vi "Install Project.vi"() -> ()   [LabVIEW 2011, in "LVH-Toolbox.lvlib" / "LVH-Build-Tools.lvlib"]
doc: "This VI will copy the source files into the install directory and create hard links replace the source files with hard links to the install directory.\n\nNote: Do not open any VI's from the source directory. All edits should be done in the Install directory to preserve paths."
uses:
  LVH-Build-Tools.lvlib
  Private/Type Defs/Install State.ctl
  Private/Type Defs/Install Configuration.ctl
  System Tools/LVH-SystemTools.lvlib
panel:
  out "Error Out":errorcluster
  out "Tab Control":enum32{"Configure", "Install", "Summary"}(tab)
  in  "Project":u16(ring) items=["lifa", "LIFCK", "LVH-EZ430-Chronos-Interface", "LVH-LINX", "LVH-Toolbox", "Traltixx"]
  in  "Install Cancel":bool
  in  "Install Next Button":bool
  in  "LabVIEW Version":u16(ring) items=["NI LabVIEW 2011 SP1", "NI LabVIEW 2013"]
  in  "Summary Finish Button":bool
  out "Source Root":string
  out "Install Root":string
  out "Components":string[](array[string])
  # "Configure"
  # "Select the project you wish to install and the LabVIEW version you wish to install to.\nClick next to continue."
  # "Installing..."
  # "Please wait while the project is installed."
  # "Summary"
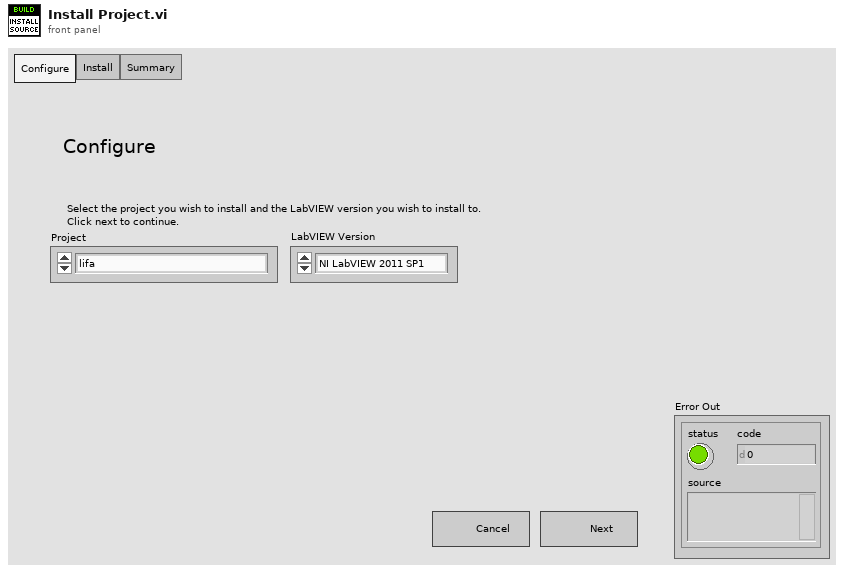
[diagram p1: front panel]
types:
  T1 = typedef "LVH-Toolbox.lvlib/LVH-Build-Tools.lvlib/Install Configuration.ctl" = cluster{"LabVIEW Directory":path, "Project Source Config":path}
  T2 = typedef "LVH-Toolbox.lvlib/LVH-Build-Tools.lvlib/Install State.ctl" = enum16{"Configure", "Install", "Summary"}
  T3 = typedef "LVH-Toolbox.lvlib/LVH-Build-Tools.lvlib/Configuration.ctl" = cluster{"Source Root":string, "Install Root":string, "Components":string[], "Ignore":string[]}
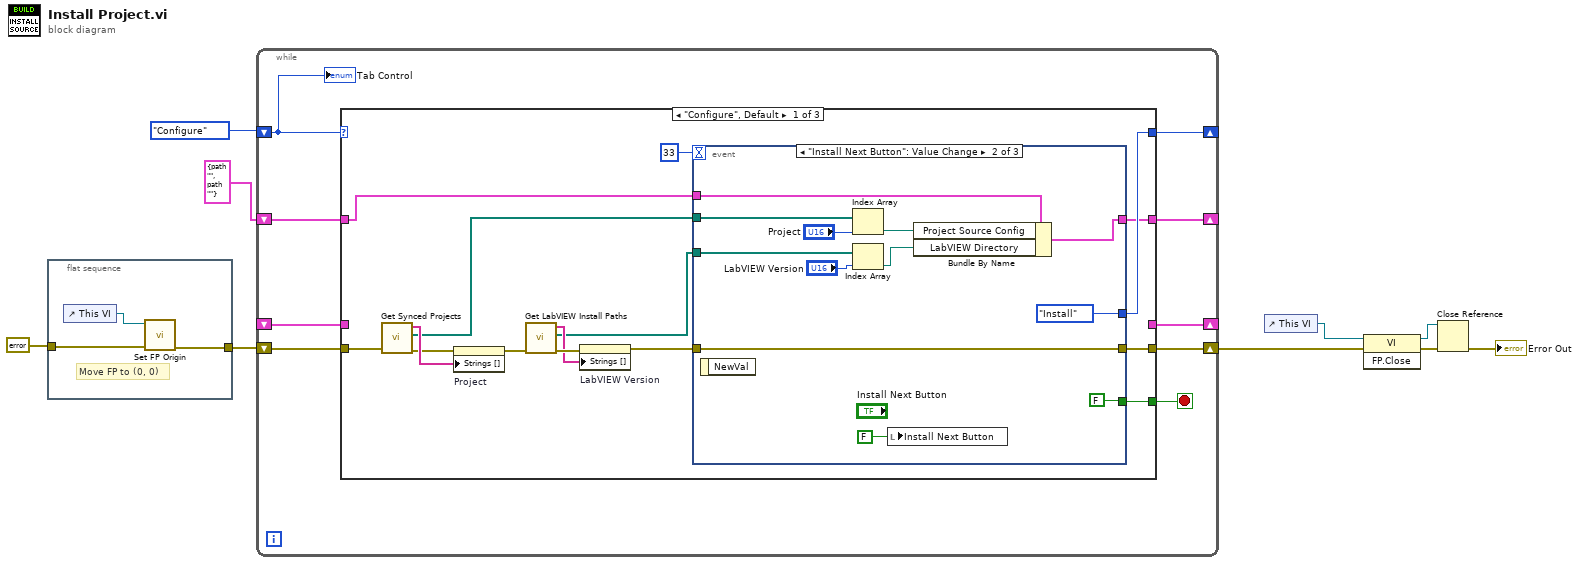
[diagram p0: block diagram]
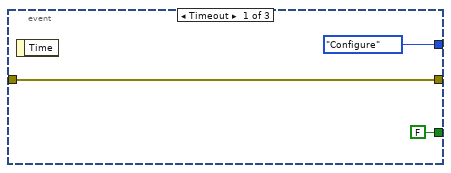
[diagram p2: hidden frame]
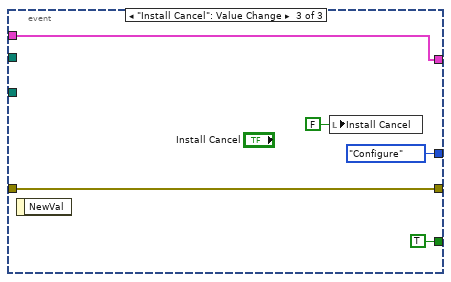
[diagram p3: hidden frame]
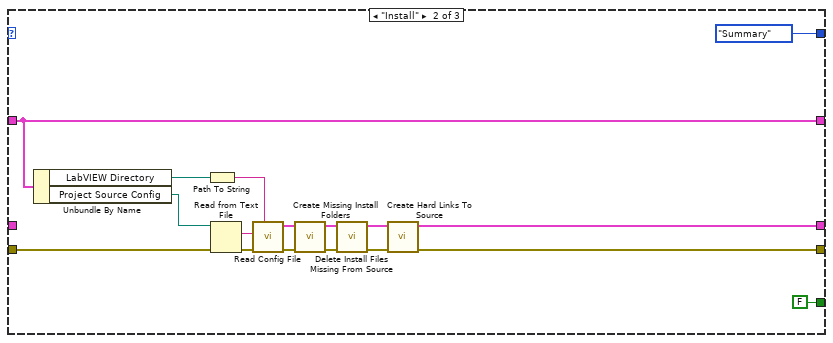
[diagram p4: hidden frame]
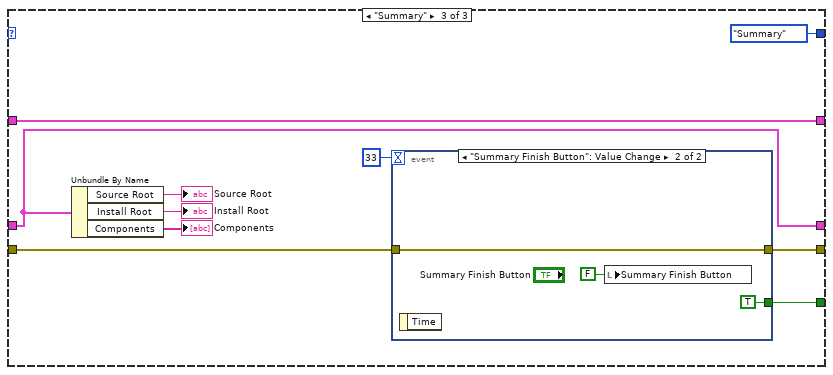
[diagram p5: hidden frame]
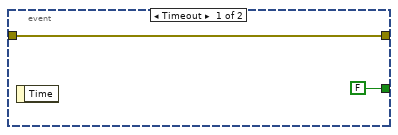
[diagram p6: hidden frame]
diagram:
  n1 = flat-sequence {
    tunnel: errorcluster {"status"=FALSE, "code"=0, "source"=""} ("Error Out") -> [w11]
    tunnel: [w10] -> w6
    frame #0 {
      # "Move FP to (0, 0)"
      n2 = control-ref of="This VI"() -> (w12:refnum<vi>)
      n3 = call "Set FP Origin.vi"("Error In"=w11, "VI Ref"=w12) -> ("Error Out"=w10:errorcluster)  [unwired: 9 in]
    }
  }
  n4 = while {
    shift-right: [w18] -> _
    shift-left: Install_State."Configure" ("Install State") -> [w19]
    shift-right: [w20] -> w4
    shift-left: w6 -> [w21]
    shift-right: [w17] -> _
    shift-left: T1 {"LabVIEW Directory"=path "", "Project Source Config"=path ""} ("Install Configuration") -> [w16]
    shift-right: [w14] -> _
    shift-left: _ -> [w13]
    stop <- w15 stop-if-true
    n5 = case shown="\"Configure\", Default" w19 {
      tunnel: w21 -> [w29 w66 w77]
      tunnel: [w33 w65 w78] -> w20
      tunnel: [w36 Install_State."Summary" ("Install State") Install_State."Summary" ("Install State")] -> w18
      tunnel: [w24 w60 w76] -> w17
      tunnel: w16 -> [w25 w60 w76]
      tunnel: [w30 FALSE w80] -> w15
      tunnel: [_ w57 w75] -> w14
      tunnel: w13 -> [_ _ w75]
      frame "Configure", Default {
        n6 = call "Get Synced Projects.vi"("Error In"=w29) -> ("Error Out"=w26:errorcluster, "Config File Paths"=w23:path[], "Synced Projects"=w28:string[])  [unwired: 8 in]
        n7 = property on="Project" class="Ring (strict)"(error in=w26, "Strings []"=w28) -> (error out=w27:errorcluster)  [unwired: 1 in, 1 out]
        n8 = call "Get LabVIEW Install Paths.vi"("Error In"=w27) -> ("Error Out"=w35:errorcluster, "Path"=w22:path[], "Version"=w34:string[])  [unwired: 8 in]
        n9 = property on="LabVIEW Version" class="Ring (strict)"(error in=w35, "Strings []"=w34) -> (error out=w32:errorcluster)  [unwired: 1 in, 1 out]
        n10 = event shown="[1] \"Install Next Button\": Value Change" {
          selector: _ -> [_ _ _]
          dyn-events: _ -> [_ _ _]
          timeout: 33 -> [_ _ _]
          tunnel: [Install_State."Configure" ("Install State") Install_State."Install" ("Install State") Install_State."Configure" ("Install State")] -> w36
          tunnel: [w38 w50 w56] -> w33
          tunnel: w32 -> [w38 w50 w56]
          tunnel: [FALSE FALSE TRUE] -> w30
          tunnel: w25 -> [_ w47 w52]
          tunnel: [_ w46 w52] -> w24
          tunnel: w23 -> [_ w44 _]
          tunnel: w22 -> [_ w42 _]
          event Timeout {
            n11 = event-data() -> ()  [unwired: 1 in, 1 out]
          }
          event "Install Next Button": Value Change {
            n12 = event-data() -> ()  [unwired: 1 in, 1 out]
            n13 = Index Array(array=w44, index="Project") -> (element=w45:path)
            n14 = Index Array(array=w42, index="LabVIEW Version") -> (element=w43:path)
            n15 = local write "Install Next Button"(FALSE ("Next Button")) -> ()
            n16 = Bundle By Name(cluster=w47, "Project Source Config"=w45, "LabVIEW Directory"=w43) -> (w46:T1)
          }
          event "Install Cancel": Value Change {
            n17 = event-data() -> ()  [unwired: 1 in, 1 out]
            n18 = local write "Install Cancel"(FALSE ("Install Cancel")) -> ()
          }
        }
      }
      frame "Install" {
        n19 = Unbundle By Name(w60) -> ("LabVIEW Directory"=w62:path, "Project Source Config"=w59:path)
        n20 = Path To String(path=w62) -> (string=w61:string)
        n21 = Read from Text File(file (use dialog)=w59, error in=w66) -> (text=w72:string, error out=w73:errorcluster)  [unwired: 2 in, 2 out]
        n22 = call "Read Config File.vi"("LabVIEW Path Override"=w61, "error in (no error)"=w73, "Config File In"=w72) -> ("error out"=w71:errorcluster, "Configuration out"=w64:T3)  [unwired: 7 in]
        n23 = call "Create Missing Install Folders.vi"("Error In"=w71, "Configuration"=w64) -> ("Error Out"=w69:errorcluster, "Configuration"=w70:T3)  [unwired: 8 in]
        n24 = call "Delete Install Files Missing From Source.vi"("Error In"=w69, "Configuration"=w70) -> ("Error Out"=w67:errorcluster, "Configuration"=w68:T3)  [unwired: 7 in, 1 out]
        n25 = call "Create Hard Links To Source.vi"("Error In"=w67, "Configuration"=w68) -> ("Error Out"=w65:errorcluster, "Configuration"=w57:T3)  [unwired: 8 in]
      }
      frame "Summary" {
        n26 = Unbundle By Name(w75) -> ("Source Root"=→"Source Root":string, "Install Root"=→"Install Root":string, "Components"=→"Components":string[])
        n27 = event shown="[1] \"Summary Finish Button\": Value Change" {
          selector: _ -> [_ _]
          dyn-events: _ -> [_ _]
          timeout: 33 -> [_ _]
          tunnel: [FALSE TRUE] -> w80
          tunnel: [w85 w86] -> w78
          tunnel: w77 -> [w85 w86]
          event Timeout {
            n28 = event-data() -> ()  [unwired: 1 in, 1 out]
          }
          event "Summary Finish Button": Value Change {
            n29 = event-data() -> ()  [unwired: 1 in, 1 out]
            n30 = local write "Summary Finish Button"(FALSE ("Summary Finish Button")) -> ()
          }
        }
      }
    }
    "Tab Control" <- w19
  }
  n31 = control-ref of="This VI"() -> (w5:refnum<vi>)
  n32 = invoke class="VI" method="FP.Close"(reference=w5, error in=w4) -> (reference out=w3:refnum<vi>, error out=w2:errorcluster)  [unwired: 1 in, 1 out]
  n33 = Close Reference(reference=w3, error in (no error)=w2) -> (error out=→"Error Out":errorcluster)
